vi "Set IConfiguration.vi"(8 "error in":errorcluster, 10 "IConfiguration":refnum<class "IConfiguration.lvclass">, 11 "Virtual PWM Generator in":refnum<class "Virtual PWM Generator.lvclass">) -> (0 "error out":errorcluster, 3 "Virtual PWM Generator out":refnum<class "Virtual PWM Generator.lvclass">)   [LabVIEW 2024, in "Virtual PWM Generator.lvclass"]
uses:
  Virtual PWM Generator.lvclass
  Source/Interfaces/IConfiguration/IConfiguration.lvclass
  Virtual PWM Generator.lvclass/Virtual PWM Generator.ctl
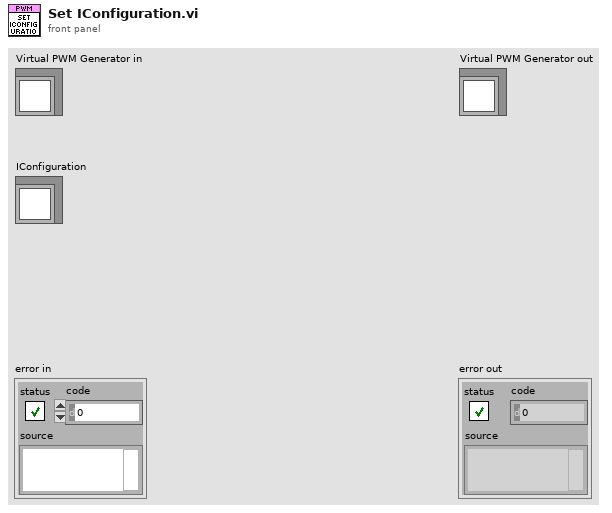
[diagram p1: front panel]
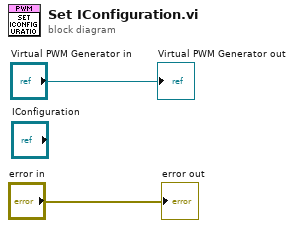
[diagram p0: block diagram]
diagram:
  "error out" <- "error in"
  "Virtual PWM Generator out" <- "Virtual PWM Generator in"
